vi "Commit Physical Channel Properties.vi"(0 "Session Handle in":T1, 5 "physical channels":refnum<k21>="$DefaultPhysChans", 11 "error in (no error)":errorcluster) -> (4 "Session Handle out":T1, 15 "error out":errorcluster)   [LabVIEW 2015, in "SLSC Switch.lvlib" / "SLSC Session.lvclass"]
uses:
  SLSC Session.lvclass
  Typedefs/Session Handle.ctl
  SLSC Session.lvclass/SLSC Session.ctl
  <vilib>/SLSC/Commit Properties for Phys Chans.vi
  <vilib>/SLSC/SLSC.lvlib
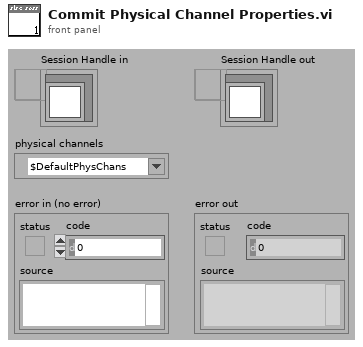
[diagram p1: front panel]
types:
  T1 = typedef "SLSC Switch.lvlib/SLSC Session.lvclass/Session Handle.ctl" = refnum<data-value>
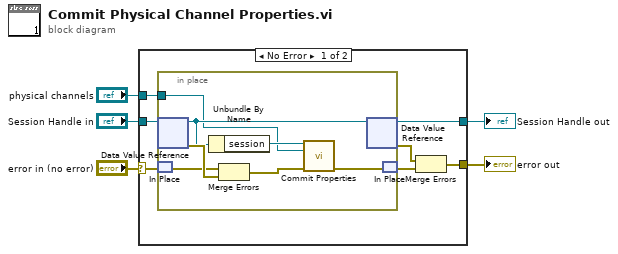
[diagram p0: block diagram]
diagram:
  n1 = case shown="No Error" "error in (no error)" {
    selector: "error in (no error)" -> [w7 w20]
    tunnel: "Session Handle in" -> [w12 w21]
    tunnel: [w11 w21] -> w4
    tunnel: [w8 w20] -> w3
    tunnel: "physical channels" -> [w6 _]
    frame No Error {
      n2 = in-place {
        in-place-border: w6 -> [w15]
        n3 = in-place-dvr #1(w12) -> (w17:refnum<class "SLSC Session.lvclass">, w19:errorcluster)
        n4 = in-place-match #2(w7) -> (w18:errorcluster)
        n5 = Unbundle By Name(w17) -> ("session"=w16:refnum<k21>)
        n6 = Merge Errors(w18, w19) -> (w14:errorcluster)
        n7 = call-poly <vilib>:"Commit Properties.vi"("session in"=w16, "physical channels"=w15, "error in (no error)"=w14) -> ("error out"=w13:errorcluster)  [unwired: 11 in, 1 out]
        n8 = in-place-dvr #1(w17) -> (w11:T1, w9:errorcluster)
        n9 = in-place-match #2(w13) -> (w10:errorcluster)
      }
      n10 = Merge Errors(w9, w10) -> (w8:errorcluster)
    }
    frame Error {
    }
  }
  "Session Handle out" <- w4
  "error out" <- w3
